vi "Spectrograph_logEvent_linearStageReportedPosition.vi"(8 "error in (no error)":errorcluster, 11 "logevent_linearStageReportedPosition_Ctl":T1) -> (0 "error out":errorcluster, 2 "function return":i32, 3 "logevent_linearStageReportedPosition_Ctl out":T1)   [LabVIEW 2016, in "SALLV_Spectrograph.lvlib"]
doc: "int Spectrograph_shm_logEvent_linearStageReportedPositionLV(Spectrograph_logevent_linearStageReportedPositionLV *logevent_linearStageReportedPosition_Ctl );"
uses:
  SALLV_Spectrograph.lvlib
  DataTypes/logevent_linearStageReportedPosition.ctl
  SALLV_Spectrograph.so
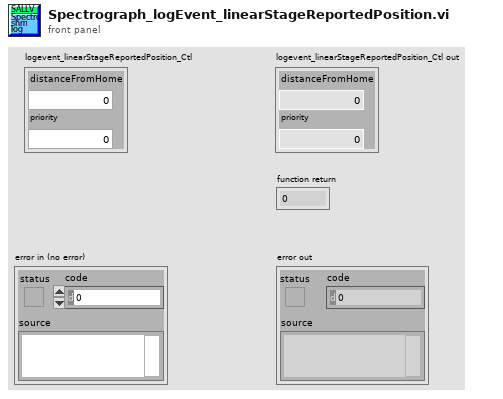
[diagram p1: front panel]
types:
  T1 = typedef "SALLV_Spectrograph.lvlib/logevent_linearStageReportedPosition.ctl" = cluster{"distanceFromHome":dbl, "priority":i32}
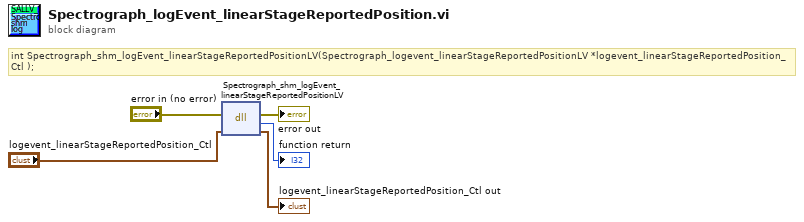
[diagram p0: block diagram]
diagram:
  # "int Spectrograph_shm_logEvent_linearStageReportedPositionLV(Spectrograph_logevent_linearStageReportedPositionLV *logevent_linearStageReportedPosition_Ctl );"
  n1 = dll-call lib="home/harini/TCS/SALLV_Spectrograph/SALLV_Spectrograph.*" fn="Spectrograph_shm_logEvent_linearStageReportedPositionLV"(error in="error in (no error)", "logevent_linearStageReportedPosition_Ctl"="logevent_linearStageReportedPosition_Ctl") -> (error out=→"error out":errorcluster, →"function return":i32, "logevent_linearStageReportedPosition_Ctl"=→"logevent_linearStageReportedPosition_Ctl out":T1)  [unwired: 2 in, 1 out]
